vi "getShutterStatus.vi"(6 "Delay between send and receive [ms]":i32=100, 8 "error in (no error)":errorcluster, 11 "Monochromator in":refnum<class "Monochromator.lvclass">) -> (0 "error out":errorcluster, 1 "shutterPosition":i32, 2 "shutterIndex":i32, 3 "Monochromator out":refnum<class "Monochromator.lvclass">)   [LabVIEW 2023, in "horiba.lvlib" / "Monochromator.lvclass"]
doc: "Returns the status of the currently selected shutter.\n\nNote: To view the status of the shutter solenoid the device must be configured for internal shutter mode.\n\nlocationId Integer. Identifies the currently selected shutter.\n0 = Shutter 1 (Front shutter)\n1 = Shutter 2 (Side shutter)\nposition Integer. Shutter position status.\n0 = Closed\n1 = Open"
uses:
  Monochromator.lvclass
  ShutterStatus.ctl
  d9b87029-586e-44ee-a6e5-d4a5e0edce38.vi
  b59fd1e7-dcda-425c-bd6c-61aafb79e7f4.vi
  <vilib>/JDP Science/JSONtext/Variant to JSON Text.vi
  <vilib>/JDP Science/JSONtext/Set Item.vi
  <vilib>/JDP Science/JSONtext/JSON text to Variant.vi
  <vilib>/JDP Science/JSONtext/LVClass Serializer/JSONtext LVClass Serializer.lvclass
  GenericDevice/GenericDevice.lvclass
panel:
  # "Connector Pane"
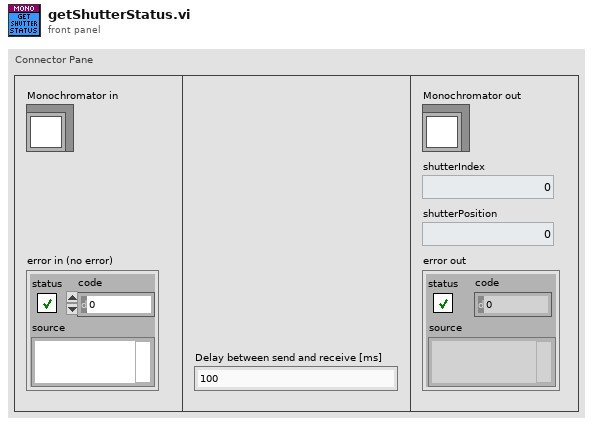
[diagram p1: front panel]
types:
  T1 = typedef "horiba.lvlib/Monochromator.lvclass/ShutterStatus.ctl" = cluster{"shutterIndex":i32, "shutterPosition":i32}
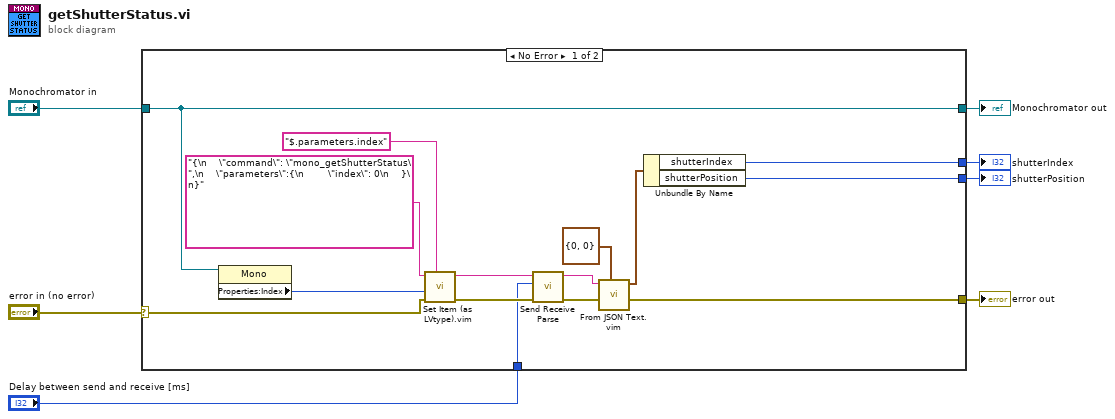
[diagram p0: block diagram]
diagram:
  n1 = case shown="No Error" "error in (no error)" {
    selector: "error in (no error)" -> [w18 w24]
    tunnel: [w17 w24] -> w6
    tunnel: [w20 w23] -> w4
    tunnel: "Monochromator in" -> [w20 w23]
    tunnel: "Delay between send and receive [ms]" -> [w12 _]
    tunnel: [w9 _] -> w2
    tunnel: [w8 _] -> w1
    frame No Error {
      n2 = property class="Mono"(reference=w20) -> ("Properties:Index"=w19:i32)  [unwired: 1 in, 2 out]
      n3 = call "Set Item (as LVtype).vim"("$Path or Item Name"="$.parameters.index", "error in (no error)"=w18, "Anything"=w19, "JSON"="{\n    \"command\": \"mono_getShutterStatus\",\n    \"parameters\":{\n        \"index\": 0\n    }\n}") -> ("error out"=w16:errorcluster, "<JSON>"=w13:string)  [unwired: 4 in, 1 out]
      n4 = call "Send Receive Parse.vi"("error in"=w16, "Delay between send and receive [ms]"=w12, "<JSON>"=w13) -> ("error out"=w14:errorcluster, "results-JSON string"=w15:string)  [unwired: 6 in, 1 out]
      n5 = call "From JSON Text.vim"("Data Type and Default Value"=T1 {"shutterIndex"=0, "shutterPosition"=0} ("Shutter Status"), "error in (no error)"=w14, "JSON"=w15) -> ("error out"=w17:errorcluster, "Data out"=w10:T1)  [unwired: 7 in]
      n6 = Unbundle By Name(w10) -> ("shutterIndex"=w9:i32, "shutterPosition"=w8:i32)
    }
    frame Error {
    }
  }
  "error out" <- w6
  "Monochromator out" <- w4
  "shutterIndex" <- w2
  "shutterPosition" <- w1
